vi "talk_to_observers.vi"(8 "error in (no error)":errorcluster, 10 "data":variant, 11 "GenericToplevelComponent in":refnum<class "GenericToplevelComponent.lvclass">) -> (0 "error out":errorcluster, 3 "GenericToplevelComponent out":refnum<class "GenericToplevelComponent.lvclass">)   [LabVIEW 2010, in "GenericToplevelComponent.lvclass"]
uses:
  GenericToplevelComponent.lvclass
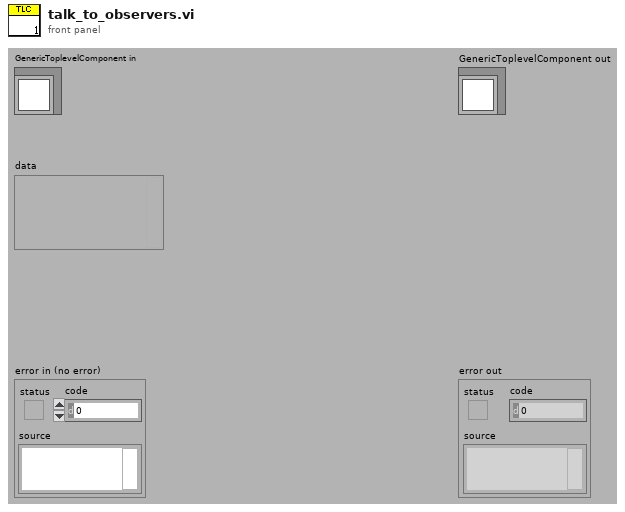
[diagram p1: front panel]
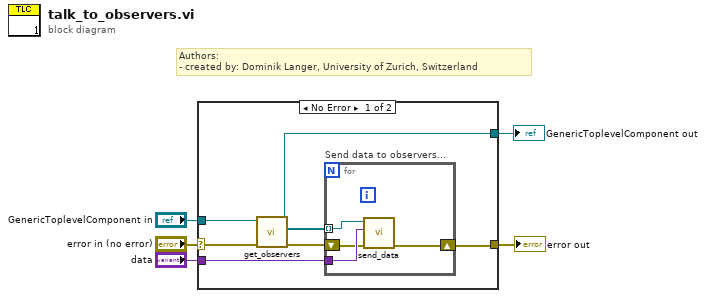
[diagram p0: block diagram]
diagram:
  # "Authors: \n- created by: Dominik Langer, University of Zurich, Switzerland"
  n1 = case shown="No Error" "error in (no error)" {
    selector: "error in (no error)" -> [w10 w18]
    tunnel: [w11 w18] -> w4
    tunnel: [w6 w17] -> w2
    tunnel: "GenericToplevelComponent in" -> [w7 w17]
    tunnel: "data" -> [w12 _]
    frame No Error {
      n2 = call-dynamic "get_observers.vi"("error in (no error)"=w10, "GenericToplevelComponent in"=w7) -> ("error out"=w9:errorcluster, "observers"=w8:refnum<class "GenericToplevelComponent.lvclass">[], "GenericToplevelComponent out"=w6:refnum<class "GenericToplevelComponent.lvclass">)  [unwired: 7 in]
      n3 = for "Send data to observers..." {
        shift-right: [w16] -> w11
        shift-left: w9 -> [w14]
        tunnel: w12 -> [w15]
        tunnel: w8 -> [w13] mode=indexing
        n4 = call-dynamic "send_data.vi"("error in (no error)"=w14, "data"=w15, "GenericToplevelComponent in"=w13) -> ("error out"=w16:errorcluster)  [unwired: 6 in, 2 out]
      }
    }
    frame Error {
    }
  }
  "error out" <- w4
  "GenericToplevelComponent out" <- w2
